vi "Write Image i16.vi"(8 "Error In":errorcluster, 10 "Data":i16[][][](array[numeric]), 11 "Image Object":T1={"Device ID"=0, "Memeroy ID"=0, "Image Parameters"={"Channel Order"=enum."CL_LUMINANCE (Grayscale)", "Dimension"={"Depth"=1, "Height"=1, "Width"=1}, "Data Type"=enum."32f", "Offset"={"X"=0, "Y"=0, "Z"=0}}} {"Image Parameters"."Dimension"."Width" min=1; "Image Parameters"."Dimension"."Height" min=1; "Image Parameters"."Dimension"."Depth" min=1}) -> (0 "Error Out":errorcluster, 3 "Image Object Out":T1={"Device ID"=0, "Memeroy ID"=0, "Image Parameters"={"Channel Order"=enum."CL_LUMINANCE (Grayscale)", "Dimension"={"Depth"=1, "Height"=1, "Width"=1}, "Data Type"=enum."32f", "Offset"={"X"=0, "Y"=0, "Z"=0}}} {"Image Parameters"."Dimension"."Width" min=1; "Image Parameters"."Dimension"."Height" min=1; "Image Parameters"."Dimension"."Depth" min=1}, 4 "Time in ms":dbl)   [LabVIEW 2012, in "OpenCLV x64.lvlib"]
doc: "Writes width by height by depth i16 data from the host to an Image Object on the device."
uses:
  OpenCLV x64.lvlib
  Controls/Image Object.ctl
  Controls/Device ID.ctl
  Controls/Memory ID.ctl
  Controls/Image Parameters.ctl
  Channel Order.ctl
  User Controls/Array Dimensions.ctl
  Data Type.ctl
  User Controls/Offset.ctl
  Error Checking/Add Error Functional Global.vi
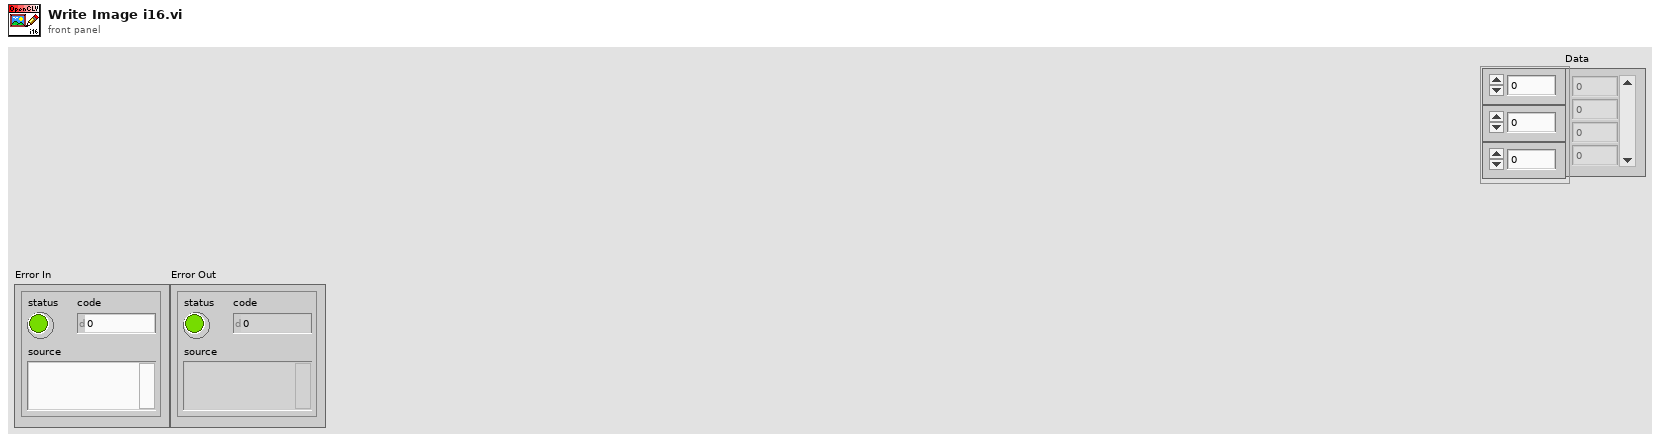
[diagram p1: front panel]
types:
  T1 = typedef "OpenCLV x64.lvlib/Image Object.ctl" = cluster{"Device ID":T2, "Memeroy ID":T3, "Image Parameters":T4}
  T2 = typedef "OpenCLV x64.lvlib/Device ID.ctl" = u64
  T3 = typedef "OpenCLV x64.lvlib/Memory ID.ctl" = u64
  T4 = typedef "OpenCLV x64.lvlib/Image Parameters.ctl" = cluster{"Channel Order":T5, "Dimension":T6, "Data Type":T7, "Offset":T8}
  T5 = typedef "OpenCLV x64.lvlib/Channel Order.ctl" = enum16{"CL_LUMINANCE (Grayscale)", "CL_INTENSITY (Opacity)", "CL_RGBA", "CL_ARGB", "CL_BGRA", "CL_RG", "CL_RA", "CL_R", "CL_A"}
  T6 = typedef "Array Dimensions.ctl" = cluster{"Depth":u64, "Height":u64, "Width":u64}
  T7 = typedef "OpenCLV x64.lvlib/Data Type.ctl" = enum16{"32f", "u8", "u16", "u32", "i8", "i16", "i32"}
  T8 = typedef "Offset.ctl" = cluster{"X":u64, "Y":u64, "Z":u64}
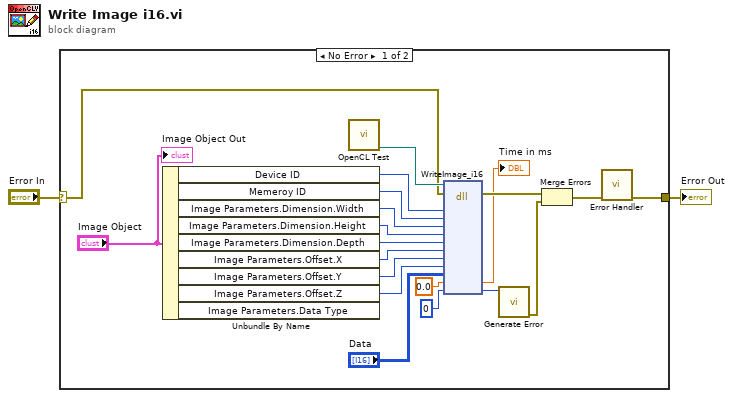
[diagram p0: block diagram]
diagram:
  n1 = case shown="No Error" "Error In" {
    selector: "Error In" -> [w3 w23]
    tunnel: [w4 w23] -> w1
    frame No Error {
      n2 = Unbundle By Name("Image Object") -> ("Device ID"=w19:T2, "Memeroy ID"=w18:T3, "Image Parameters.Dimension.Width"=w17:u64, "Image Parameters.Dimension.Height"=w16:u64, "Image Parameters.Dimension.Depth"=w15:u64, "Image Parameters.Offset.X"=w13:u64, "Image Parameters.Offset.Y"=w12:u64, "Image Parameters.Offset.Z"=w11:u64)  [unwired: 1 out]
      n3 = call "OpenCL Test.vi"() -> ("DLL To Use"=w6:path)  [unwired: 11 in]
      n4 = dll-call lib="C:/Users/bme-amcelroy-la/Desktop/OpenCLV/trunk/OpenCLV_x64_1.0/OpenCLV_x64.dll" fn="WriteImage_i16"(path in=w6, error in=w3, "Labview Device"=w19, "Device Memory"=w18, "Width"=w17, "Height"=w16, "Depth"=w15, "X Offset"=w13, "Y Offset"=w12, "Z Offset"=w11, "Data"="Data", "Time in ms"=0.0, "Error"=0) -> (error out=w20:errorcluster, "Time in ms"=→"Time in ms":dbl, "Error"=w22:i32)  [unwired: 11 in, 1 out]
      n5 = call "Generate Error.vi"("Error"=w22) -> ("error out"=w21:errorcluster)  [unwired: 10 in]
      n6 = Merge Errors(w20, w21) -> (w5:errorcluster)
      n7 = call-poly "Error Handler.vi"("Error In"=w5) -> ("Error Out"=w4:errorcluster)  [unwired: 10 in]
      "Image Object Out" <- "Image Object"
    }
    frame Error {
    }
  }
  "Error Out" <- w1
